vi "Axis Conditioning.vi"(8 "rate limit (val/sec)":dbl=0.04, 10 "limit":dbl=0.04, 11 "joystick axes":dbl[](array[numeric])) -> (0 "rate limited":dbl[](array[numeric]), 3 "deadbanded":dbl[](array[numeric]))   [LabVIEW 2026]
doc: "This VI conditions axis values with\n* deadband -- forcing small values to zero\n* rate limiting -- controlling how quickly the value can change over time"
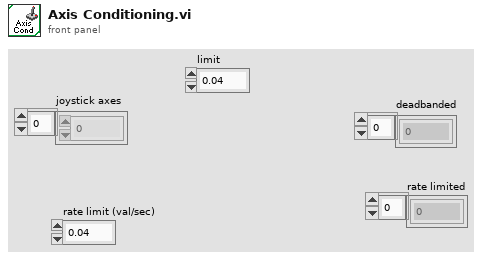
[diagram p1: front panel]
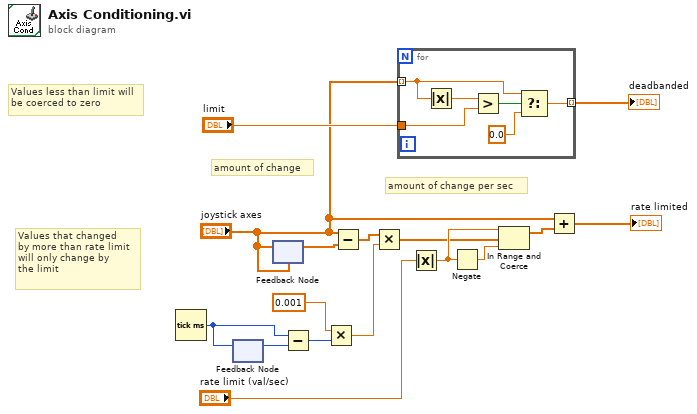
[diagram p0: block diagram]
diagram:
  # "amount of change per sec"
  # "Values that changed\nby more than rate limit\nwill only change by\nthe limit"
  # "Values less than limit will\nbe coerced to zero"
  # "amount of change"
  n1 = Tick Count (ms)() -> (millisecond timer value=w6:u32)
  n2 = feedback #1() -> (w5:u32)  [unwired: 1 in]
  n3 = feedback-in #1(w6) -> ()
  n4 = feedback-in #2("joystick axes") -> ()
  n5 = feedback #2("joystick axes") -> (w16:dbl[])
  n6 = Subtract(x=w6, y=w5) -> (x-y=w3:u32)
  n7 = Multiply(x=0.001, y=w3) -> (x*y=w2:dbl)
  n8 = Subtract(x="joystick axes", y=w16) -> (x-y=w15:dbl[])
  n9 = Multiply(x=w15, y=w2) -> (x*y=w4:dbl[])
  n10 = for {
    tunnel: "limit" -> [w22]
    tunnel: "joystick axes" -> [w17] mode=indexing
    tunnel: [w19] -> w8 mode=indexing
    n11 = Absolute Value(x=w17) -> (abs(x)=w18:dbl)
    n12 = Greater?(x=w18, y=w22) -> (0:w21:bool)
    n13 = Select(t=w17, s=w21, f=0.0) -> (s? t:f=w19:dbl)
  }
  "deadbanded" <- w8
  n14 = Absolute Value(x="rate limit (val/sec)") -> (abs(x)=w13:dbl)
  n15 = Negate(x=w13) -> (-x=w12:dbl)
  n16 = In Range and Coerce(upper limit=w13, x=w4, lower limit=w12) -> (coerced(x)=w11:dbl[])  [unwired: 1 out]
  n17 = Add(x="joystick axes", y=w11) -> (x+y=→"rate limited":dbl[])
